vi "Register UI user events.vi"(8 "error in (no error)":errorcluster, 11 "Execution UI In":refnum<class "Execution UI V2.lvclass">) -> (0 "error out":errorcluster, 2 "Event Registration Refnum":refnum<event-registration>, 3 "Execution UI Out":refnum<class "Execution UI V2.lvclass">)   [LabVIEW 2020, in "Execution UI V2.lvclass"]
uses:
  Execution UI V2.lvclass
  Execution UI V2.lvclass/Execution UI V2.ctl
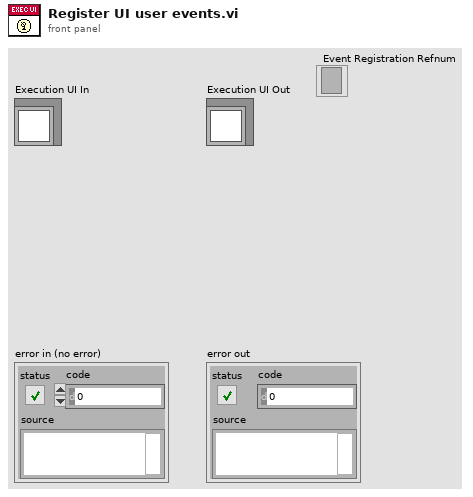
[diagram p1: front panel]
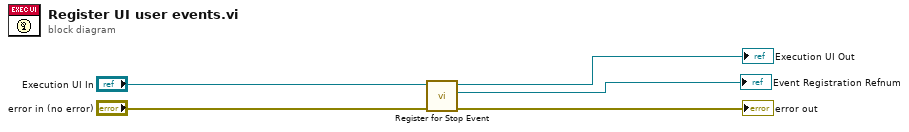
[diagram p0: block diagram]
diagram:
  n1 = call "Register for Stop Event.vi"("error in (no error)"="error in (no error)", "Execution UI In"="Execution UI In") -> ("error out"=→"error out":errorcluster, "Event Registration Refnum"=→"Event Registration Refnum":refnum<event-registration>, "Execution UI Out"=→"Execution UI Out":refnum<class "Execution UI V2.lvclass">)  [unwired: 7 in]
